vi "Ultima aula.vi"() -> ()   [LabVIEW 2024]
uses:
  <vilib>/Instr/_visa.llb/VISA Configure Serial Port (Instr).vi
panel:
  out "output 2":dbl
  out "Waveform Chart 2":dbl(graph)
  out "Waveform Chart":dbl(graph)
  out "output 1":dbl
  in  "termination char\n(0xA = '\\n' = LF)":u8=10 format="%.0x"
  out "read buffer":string
  in  "operation":dbl
  in  "stop":bool
  in  "VISA resource name":refnum<visa-resource-name>
  in  "write buffer":string
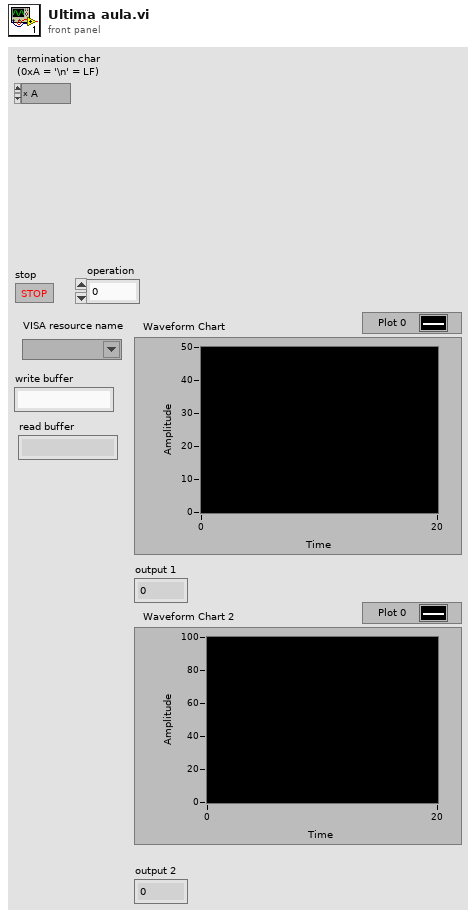
[diagram p1: front panel]
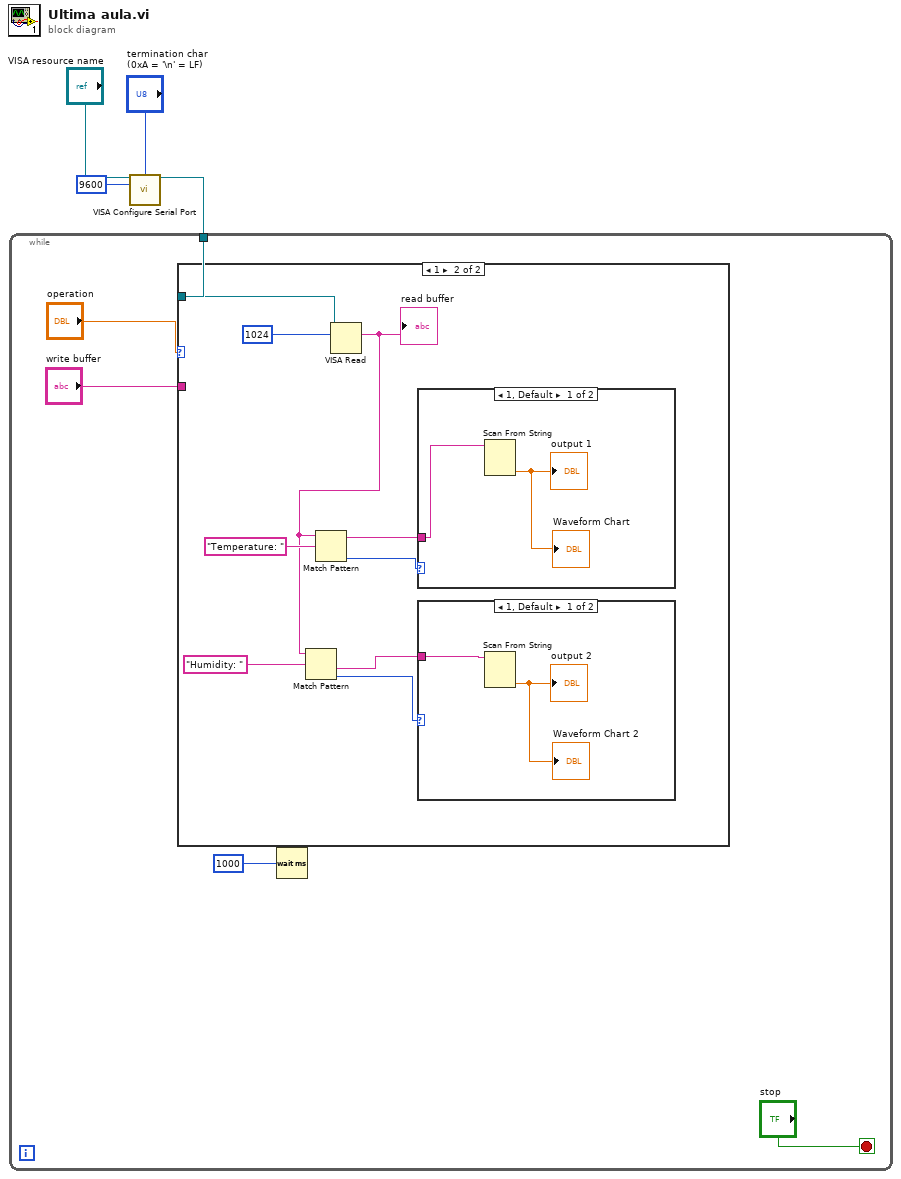
[diagram p0: block diagram]
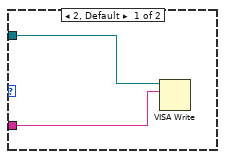
[diagram p2: hidden frame]
diagram:
  n1 = call-poly "VISA Configure Serial Port"("VISA resource name"="VISA resource name", "termination char\n(0xA = '\\n' = LF)"="termination char\n(0xA = '\\n' = LF)", "baud rate (9600)"=u32 9600) -> ("VISA resource name out"=w3:refnum<visa-resource-name>)  [unwired: 11 in, 1 out]
  n2 = while {
    tunnel: w3 -> [w6]
    stop <- "stop" stop-if-true
    n3 = case shown="1" "operation" {
      tunnel: "write buffer" -> [w11 _]
      tunnel: w6 -> [w10 w20]
      frame 2, Default {
        n4 = VISA Write(VISA resource name=w10, write buffer=w11) -> ()  [unwired: 1 in, 3 out]
      }
      frame 1 {
        n5 = VISA Read(VISA resource name=w20, byte count=u32 1024) -> (read buffer=w12:string)  [unwired: 1 in, 3 out]
        "read buffer" <- w12
        n6 = Match Pattern(string=w12, regular expression="Humidity: ") -> (after substring=w15:string, offset past match=w14:i32)  [unwired: 1 in, 2 out]
        n7 = Match Pattern(string=w12, regular expression="Temperature: ") -> (after substring=w17:string, offset past match=w13:i32)  [unwired: 1 in, 2 out]
        n8 = case shown="1, Default" w13 {
          tunnel: w17 -> [w24 _]
          frame 1, Default {
            n9 = Scan From String(input string=w24) -> (output 1=→"output 1" →"Waveform Chart":dbl)  [unwired: 4 in, 3 out]
          }
          frame 2 {
          }
        }
        n10 = case shown="1, Default" w14 {
          tunnel: w15 -> [w22 _]
          frame 1, Default {
            n11 = Scan From String(input string=w22) -> (output 1=→"output 2" →"Waveform Chart 2":dbl)  [unwired: 4 in, 3 out]
          }
          frame 2 {
          }
        }
      }
    }
    n12 = Wait (ms)(milliseconds to wait=u32 1000) -> ()  [unwired: 1 out]
  }
